vi "marshalling.vi"(8 "error in (no error)":errorcluster, 10 "Variant":variant, 11 "Serializer":refnum<class "Serializer.PlainText.lvclass">) -> (0 "error out":errorcluster, 2 "String":string, 3 "Serializer out":refnum<class "Serializer.PlainText.lvclass">)   [LabVIEW 2013, in "OpenSerializer.lvlib" / "Serializer.PlainText.lvclass"]
uses:
  Serializer.PlainText.lvclass
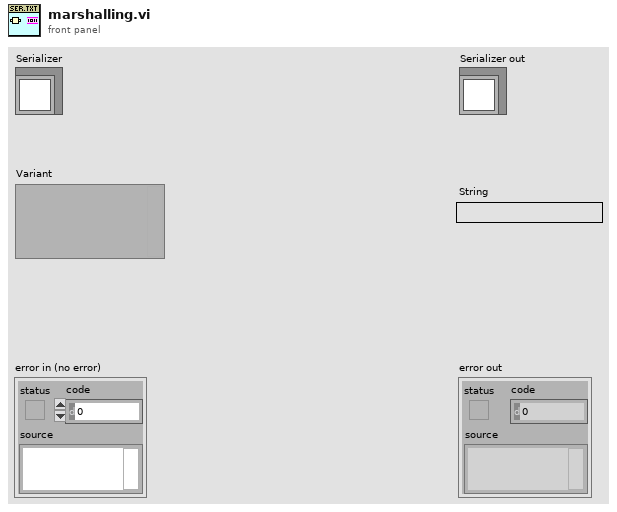
[diagram p1: front panel]
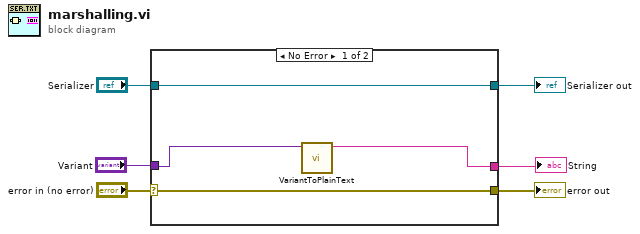
[diagram p0: block diagram]
diagram:
  n1 = case shown="No Error" "error in (no error)" {
    selector: "error in (no error)" -> [w9 w12]
    tunnel: [w9 w12] -> w5
    tunnel: [w10 w11] -> w3
    tunnel: "Serializer" -> [w10 w11]
    tunnel: "Variant" -> [w8 _]
    tunnel: [w7 _] -> w1
    frame No Error {
      n2 = call "VariantToPlainText.vi"("Variant-formatted Value"=w8) -> ("String-formatted Value"=w7:string)  [unwired: 10 in]
    }
    frame Error {
    }
  }
  "error out" <- w5
  "Serializer out" <- w3
  "String" <- w1
